vi "Disabled.vi"(7 "Robot Mode":T2, 10 "Match Info":T1={"Autonomous Elapsed Seconds"=0.0, "TeleOp Elapsed Seconds"=0.0, "Disabled Elapsed Seconds"=0.0, "Visited Autonomous"=FALSE, "Visited TeleOp"=FALSE, "Visited Disabled"=FALSE, "Autonomous Settings"={"Autonomous Style"=enum."Independent", "VI Refnum"=refnum}}, 11 "Call Context":T3) -> ()   [LabVIEW 2012]
doc: "This VI is called each time a disabled packet is received from the DS. It is often used to prepare for the next robot mode, to calibrate sensors, etc."
uses:
  <vilib>/Rock Robotics/WPI/DriverStation/WPI_DriverStationDerivedRobotMode.ctl
  <vilib>/Rock Robotics/WPI/DriverStation/WPI_DriverStationRobotMode2.ctl
  <vilib>/Rock Robotics/WPI/DriverStation/WPI_DriverStationMatch Info.ctl
  Robot Global Data.vi
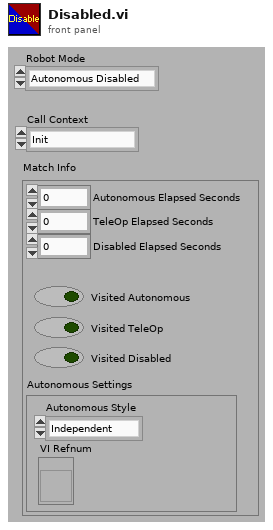
[diagram p1: front panel]
types:
  T1 = typedef "WPI_DriverStationMatch Info.ctl" = cluster{"Autonomous Elapsed Seconds":dbl, "TeleOp Elapsed Seconds":dbl, "Disabled Elapsed Seconds":dbl, "Visited Autonomous":bool, "Visited TeleOp":bool, "Visited Disabled":bool, "Autonomous Settings":cluster{"Autonomous Style":enum16{"Iterative", "Independent"}, "VI Refnum":refnum<vi>}}
  T2 = typedef "WPI_DriverStationRobotMode2.ctl" = enum16{"Autonomous Disabled", "Autonomous Enabled", "Teleop Disabled", "Teleop Enabled", "Timeout", "Finish", "Test Disabled", "Test Enabled"}
  T3 = typedef "WPI_DriverStationDerivedRobotMode.ctl" = enum16{"Init", "Execute", "Stop"}
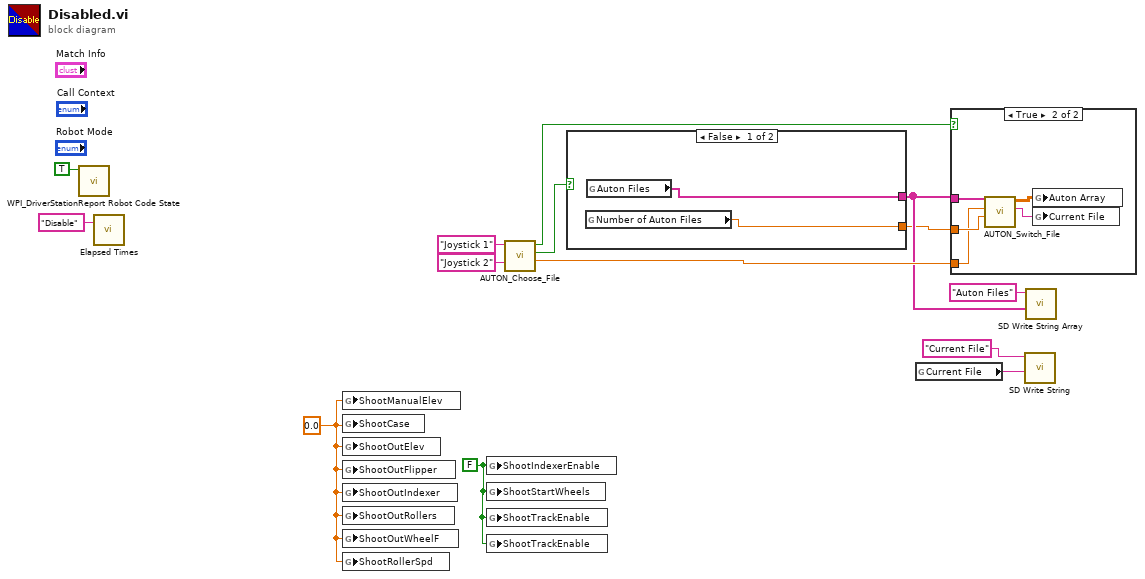
[diagram p0: block diagram]
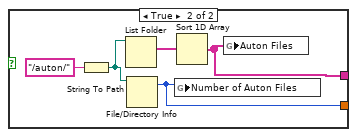
[diagram p3: hidden frame]
diagram:
  w2 = FALSE ("ShootIndexerEnable")
  w1 = 0.0 ("ShootCase")
  n1 = call <vilib>:"WPI_DriverStationReport Robot Code State.vi"("Disabled"=TRUE ("Autonomous")) -> ()  [unwired: 10 in, 1 out]
  n2 = call "Elapsed Times.vi"("Call Name"="Disable") -> ()  [unwired: 2 in, 1 out]
  n3 = global write "Robot Global Data.vi" "ShootManualElev"(w1) -> ()
  n4 = global write "Robot Global Data.vi" "ShootCase"(w1) -> ()
  n5 = global write "Robot Global Data.vi" "ShootOutElev"(w1) -> ()
  n6 = global write "Robot Global Data.vi" "ShootOutFlipper"(w1) -> ()
  n7 = global write "Robot Global Data.vi" "ShootOutIndexer"(w1) -> ()
  n8 = global write "Robot Global Data.vi" "ShootOutRollers"(w1) -> ()
  n9 = global write "Robot Global Data.vi" "ShootOutWheelF"(w1) -> ()
  n10 = global write "Robot Global Data.vi" "ShootRollerSpd"(w1) -> ()
  n11 = global write "Robot Global Data.vi" "ShootIndexerEnable"(w2) -> ()
  n12 = global write "Robot Global Data.vi" "ShootStartWheels"(w2) -> ()
  n13 = global write "Robot Global Data.vi" "ShootTrackEnable"(w2) -> ()
  n14 = global write "Robot Global Data.vi" "ShootTrackEnable"(w2) -> ()
  n15 = call "AUTON_Choose_File.vi"("Joystick 2 Refnum"="Joystick 2", "Joystick 1 Refnum"="Joystick 1") -> ("Auton File"=w11:dbl, "Refresh"=w10:bool, "Allow Change"=w9:bool)  [unwired: 7 in]
  n16 = case shown="False" w10 {
    tunnel: [w15 w18] -> w6
    tunnel: [w16 w17] -> w8
    frame False {
      n17 = global read "Robot Global Data.vi" "Number of Auton Files"() -> (w15:dbl)
      n18 = global read "Robot Global Data.vi" "Auton Files"() -> (w16:string[])
    }
    frame True {
      n19 = String To Path(string="/auton/") -> (path=w20:path)
      n20 = List Folder(path=w20) -> (filenames=w19:string[])  [unwired: 3 in, 3 out]
      n21 = File/Directory Info(path=w20) -> (size=w18:i64)  [unwired: 1 in, 6 out]
      n22 = global write "Robot Global Data.vi" "Number of Auton Files"(w18) -> ()
      n23 = Sort 1D Array(array=w19) -> (sorted array=w17:string[])
      n24 = global write "Robot Global Data.vi" "Auton Files"(w17) -> ()
    }
  }
  n25 = global read "Robot Global Data.vi" "Current File"() -> (w5:string)
  n26 = case shown="True" w9 {
    tunnel: w11 -> [_ w24]
    tunnel: w8 -> [_ w26]
    tunnel: w6 -> [_ w25]
    frame False {
    }
    frame True {
      n27 = call "AUTON_Switch_File.vi"("Number of Auton Files"=w25, "Auton File"=w24, "Auton Files"=w26) -> ("Current File"=w23:string, "Auton Array"=w22:dbl[][])  [unwired: 7 in]
      n28 = global write "Robot Global Data.vi" "Auton Array"(w22) -> ()
      n29 = global write "Robot Global Data.vi" "Current File"(w23) -> ()
    }
  }
  n30 = call <vilib>:"SD Write String.vi"("String"=w5, "Name"="Current File") -> ()  [unwired: 8 in, 2 out]
  n31 = call <vilib>:"SD Write String Array.vi"("String Array"=w8, "Name"="Auton Files") -> ()  [unwired: 8 in, 2 out]
